vi "AddStartEndPointsGrid.vi"(4 "Xgoal":dbl format="%#_13g", 5 "Xstart":dbl format="%#_13g", 6 "GridParameter":dbl, 7 "Ystart":dbl format="%#_13g", 8 "n vertical":dbl, 9 "Ygoal":dbl format="%#_13g", 10 "n horizontal":dbl, 11 "grid in":T1) -> (0 "Nó goal":dbl[](array[numeric]), 1 "Nó start":dbl[](array[numeric]), 2 "grid out":T1)   [LabVIEW 2016]
uses:
  grid.ctl
  elementGrid.ctl
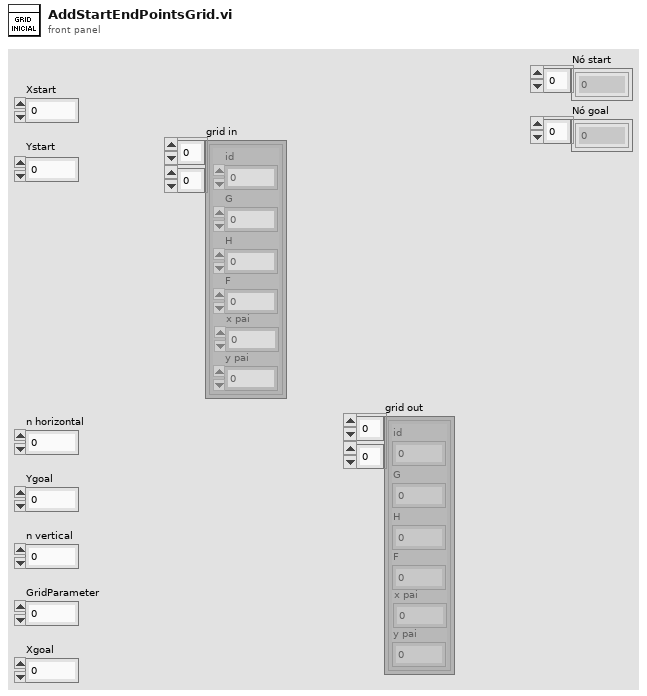
[diagram p1: front panel]
types:
  T1 = typedef "grid.ctl" = T2[][]
  T2 = typedef "elementGrid.ctl" = cluster{"id":dbl, "G":dbl, "H":dbl, "F":dbl, "x pai":dbl, "y pai":dbl}
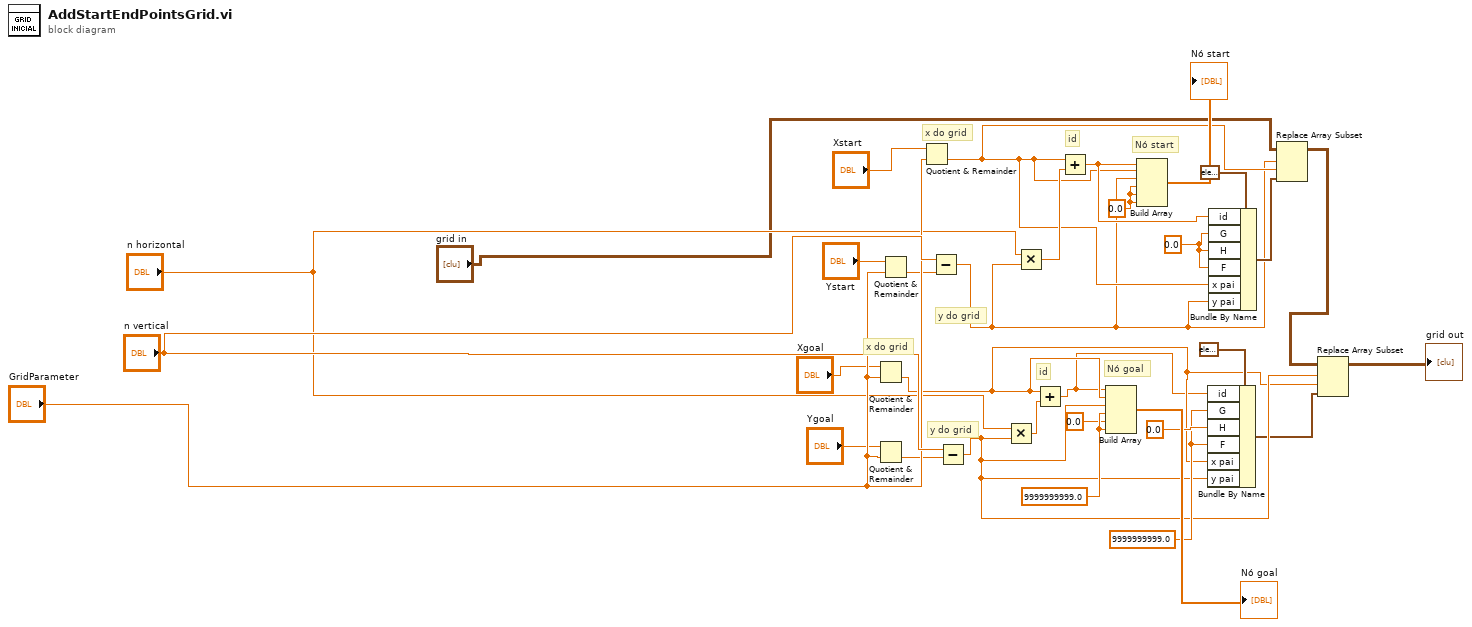
[diagram p0: block diagram]
diagram:
  w29 = 9999999999.0
  w5 = 9999999999.0
  w11 = 0.0 ("element")
  w27 = 0.0 ("element")
  # "Nó goal"
  # "Nó start"
  # "id"
  # "y do grid"
  # "x do grid"
  # "id"
  # "y do grid"
  # "x do grid"
  n1 = Quotient & Remainder(x="Xgoal", y="GridParameter") -> (floor(x/y)=w2:dbl)  [unwired: 1 out]
  n2 = Quotient & Remainder(x="Ygoal", y="GridParameter") -> (floor(x/y)=w24:dbl)  [unwired: 1 out]
  n3 = Quotient & Remainder(x="Ystart", y="GridParameter") -> (floor(x/y)=w20:dbl)  [unwired: 1 out]
  n4 = Quotient & Remainder(x="Xstart", y="GridParameter") -> (floor(x/y)=w9:dbl)  [unwired: 1 out]
  n5 = Subtract(x="n vertical", y=w20) -> (x-y=w8:dbl)
  n6 = Subtract(x="n vertical", y=w24) -> (x-y=w4:dbl)
  n7 = Multiply(x="n horizontal", y=w4) -> (x*y=w25:dbl)
  n8 = Multiply(x="n horizontal", y=w8) -> (x*y=w21:dbl)
  n9 = Add(x=w2, y=w25) -> (x+y=w1:dbl)
  n10 = Add(x=w9, y=w21) -> (x+y=w10:dbl)
  n11 = Build Array(w1, w2, w4, w29, 0.0 ("element"), w29) -> (→"Nó goal":dbl[])
  n12 = Build Array(w10, w9, w8, w27, w27, w27) -> (→"Nó start":dbl[])
  n13 = Bundle By Name(cluster=T2 {"id"=0.0, "G"=0.0, "H"=0.0, "F"=0.0, "x pai"=0.0, "y pai"=0.0} ("element"), "id"=w1, "G"=w5, "H"=0.0 ("element"), "F"=w5, "x pai"=w2, "y pai"=w4) -> (w3:T2)
  n14 = Bundle By Name(cluster=T2 {"id"=0.0, "G"=0.0, "H"=0.0, "F"=0.0, "x pai"=0.0, "y pai"=0.0} ("element"), "id"=w10, "G"=w11, "H"=w11, "F"=w11, "x pai"=w9, "y pai"=w8) -> (w12:T2)
  n15 = Replace Array Subset(array="grid in", new element=w12, index (row)=w8, index (col)=w9) -> (w28:T1)
  n16 = Replace Array Subset(array=w28, new element=w3, index (row)=w4, index (col)=w2) -> (→"grid out":T1)
